vi "Process_Directions.vi"(10 "conNum":u8[](array[numeric]), 11 "ioStatus":T1[](array[typedef])) -> (1 "OutputIndex":i32[](array[numeric]), 2 "InputIndex":i32[](array[numeric]), 3 "Directions":T1[](array[typedef]))   [LabVIEW 2020]
uses:
  <vilib>/AppBuilder/IOStatus.ctl
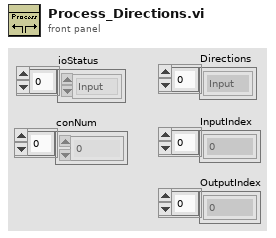
[diagram p1: front panel]
types:
  T1 = typedef "IOStatus.ctl" = enum16{"Input", "Output", "Input/Output", "InputDeleted", "OutputDeleted", "IODeleted", "ErrorClusterIn", "ErrorClusterOut"}
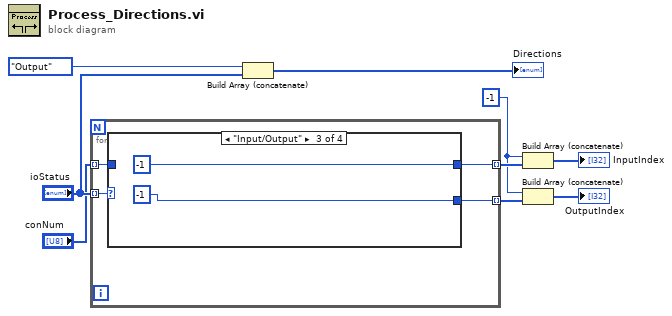
[diagram p0: block diagram]
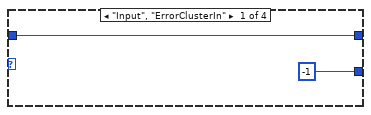
[diagram p2: hidden frame]
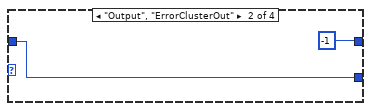
[diagram p3: hidden frame]
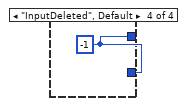
[diagram p4: hidden frame]
diagram:
  w3 = -1
  n1 = for {
    tunnel: "ioStatus" -> [w13] mode=indexing
    tunnel: "conNum" -> [w12] mode=indexing
    tunnel: [w11] -> w4 mode=indexing
    tunnel: [w10] -> w2 mode=indexing
    n2 = case shown="\"Input/Output\"" w13 {
      tunnel: w12 -> [w14 w17 _ _]
      tunnel: [w14 -1 -1 w20] -> w11
      tunnel: [-1 w17 -1 w20] -> w10
      frame "Input", "ErrorClusterIn" {
      }
      frame "Output", "ErrorClusterOut" {
      }
      frame "Input/Output" {
      }
      frame "InputDeleted", Default {
        w20 = -1
      }
    }
  }
  n3 = Build Array (concatenate)(IOStatus."Output" ("Input/Output"), "ioStatus") -> (→"Directions":T1[])
  n4 = Build Array (concatenate)(w3, w4) -> (→"InputIndex":i32[])
  n5 = Build Array (concatenate)(w3, w2) -> (→"OutputIndex":i32[])
